vi "TurboMotor.vi"() -> ()   [LabVIEW 2011]
panel:
  in  "Attribute Message Types":u16(ring) items=["Position Control Supervisor"=26, "Position Controller"=27]
  in  "Position Controller Supervisor":u16(ring) items=["Number of Attributes"=1, "Attribute List"=2, "Mode"=3, "Target Position"=6, "Target Velocity"=7, "Acceleration"=8, "Incremental Position Flag"=10, "Load Data/Start Profile/Profile in Progress"=11, "Actual Position"=13, "Actual Velocity"=14, "Commanded Position"=15, "Commanded Velocity"=16, "Enable"=17, "Smooth Stop"=20, "Hard Stop"=21, "Direction"=23, "Reference Direction"=24, "Torque"=25, "Wrap Around"=29, "Kp"=30, "Ki"=31, "Kd"=32, "MaxKi"=33, "Velocity Feed Forward"=35, "Sample Rate"=37, "Feedback Resolution"=40, ""=41, ""=42, ""=43, ""=44, "Max Dynamic Following Error"=45, "Following Error Fault"=47, "Actual Following Error"=48, "Hard Limit Action"=49, "Forward Limit"=50, "Reverse Limit"=51, "Soft Limits Enable"=52, "Soft Limit Action"=53, "Positive Soft Limit Position"=54, "Negative Soft Limit Position"=55, "Positive Limit Triggered"=56, "Negative Limit Triggered"=57, "Load Data Complete"=58, "Current Limit"=100, "Reset Motor Faults"=101, "Reset Motor"=102, "Overheat Setpoint"=103, "Temperature"=104, "Variable u"=105, "Variable v"=106, "Variable w"=107, "Variable x"=108, "GOSUBnnn"=109, "Loss of Network Action"=110, "Status Word"=111]
  in  "stop":bool
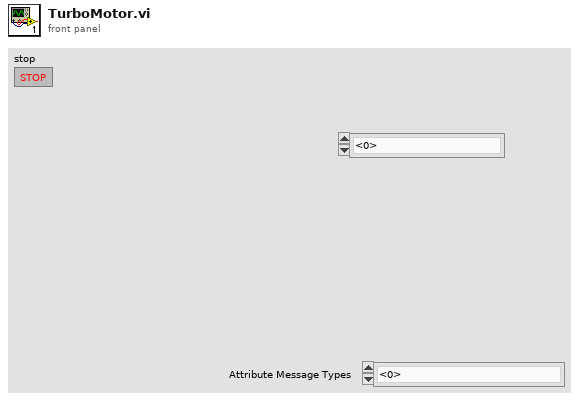
[diagram p1: front panel]
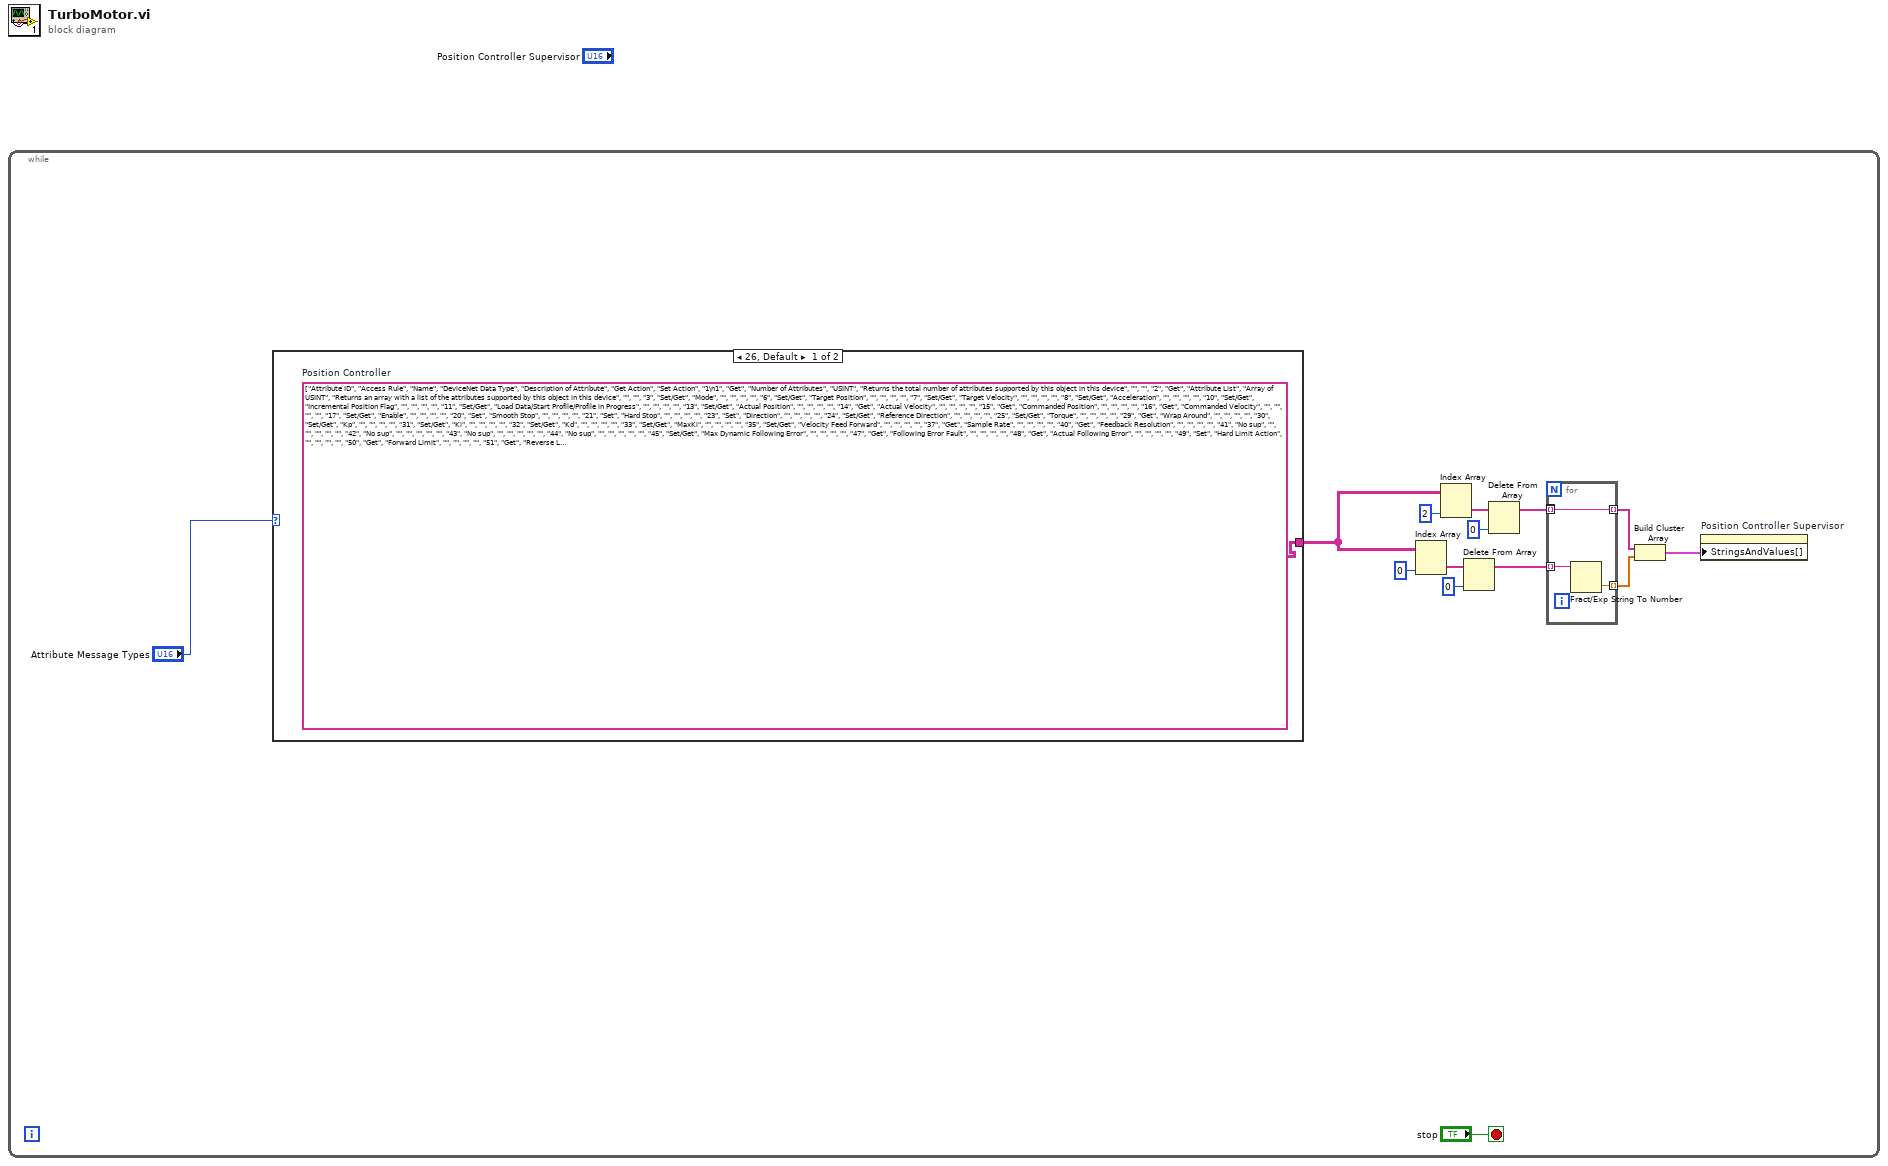
[diagram p0: block diagram]
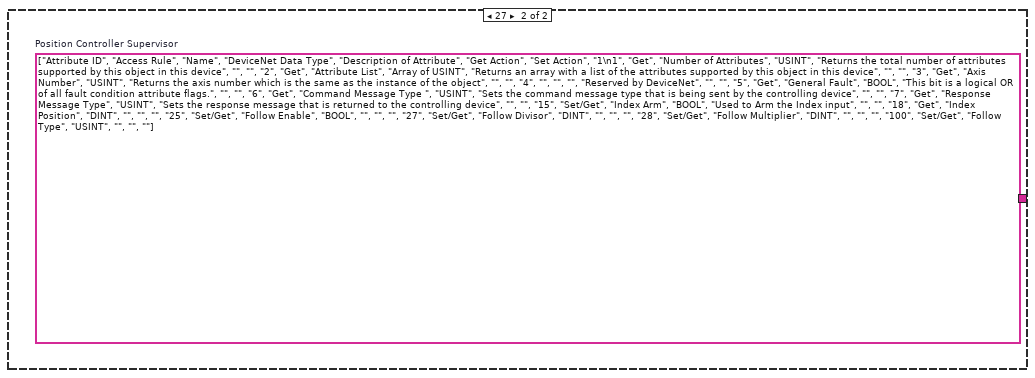
[diagram p2: hidden frame]
diagram:
  n1 = while {
    stop <- "stop" stop-if-true
    n2 = case shown="26, Default" "Attribute Message Types" {
      tunnel: [w15 w16] -> w3
      frame 26, Default {
        w15 = string[][] [["Attribute ID", "Access Rule", "Name", "DeviceNet Data Type", "Description of Attribute", "Get Action", "Set Action"], ["1\n1", "Get", "Number of Attributes", "USINT", "Returns the total number of attributes supported by this object in this device", "", ""], ["2", "Get", "Attribute List", "Array of USINT", "Returns an array with a list of the attributes supported by this object in this device", "", ""], ["3", "Set/Get", "Mode", "", "", "", ""], ["6", "Set/Get", "Target Position", "", "", "", ""], ["7", "Set/Get", "Target Velocity", "", "", "", ""], ["8", "Set/Get", "Acceleration", "", "", "", ""], ["10", "Set/Get", "Incremental Position Flag", "", "", "", ""], ["11", "Set/Get", "Load Data/Start Profile/Profile in Progress", "", "", "", ""], ["13", "Set/Get", "Actual Position", "", "", "", ""], ["14", "Get", "Actual Velocity", "", "", "", ""], ["15", "Get", "Commanded Position", "", "", "", ""], ["16", "Get", "Commanded Velocity", "", "", "", ""], ["17", "Set/Get", "Enable", "", "", "", ""], ["20", "Set", "Smooth Stop", "", "", "", ""], ["21", "Set", "Hard Stop", "", "", "", ""], ["23", "Set", "Direction", "", "", "", ""], ["24", "Set/Get", "Reference Direction", "", "", "", ""], ["25", "Set/Get", "Torque", "", "", "", ""], ["29", "Get", "Wrap Around", "", "", "", ""], ["30", "Set/Get", "Kp", "", "", "", ""], ["31", "Set/Get", "Ki", "", "", "", ""], ["32", "Set/Get", "Kd", "", "", "", ""], ["33", "Set/Get", "MaxKi", "", "", "", ""], ["35", "Set/Get", "Velocity Feed Forward", "", "", "", ""], ["37", "Get", "Sample Rate", "", "", "", ""], ["40", "Get", "Feedback Resolution", "", "", "", ""], ["41", "No sup", "", "", "", "", ""], ["42", "No sup", "", "", "", "", ""], ["43", "No sup", "", "", "", "", ""], ["44", "No sup", "", "", "", "", ""], ["45", "Set/Get", "Max Dynamic Following Error", "", "", "", ""], ["47", "Get", "Following Error Fault", "", "", "", ""], ["48", "Get", "Actual Following Error", "", "", "", ""], ["49", "Set", "Hard Limit Action", "", "", "", ""], ["50", "Get", "Forward Limit", "", "", "", ""], ["51", "Get", "Reverse Limit", "", "", "", ""], ["52", "Set/Get", "Soft Limits Enable", "", "", "", ""], ["53", "Set/Get", "Soft Limit Action", "", "", "", ""], ["54", "Set/Get", "Positive Soft Limit Position", "", "", "", ""], ["55", "Set/Get", "Negative Soft Limit Position", "", "", "", ""], ["56", "Get", "Positive Limit Triggered", "", "", "", ""], ["57", "Get", "Negative Limit Triggered", "", "", "", ""], ["58", "Get", "Load Data Complete", "", "", "", ""], ["100", "Set", "Current Limit", "", "", "", ""], ["101", "Set", "Reset Motor Faults", "", "", "", ""], ["102", "Set", "Reset Motor", "", "", "", ""], ["103", "Set/Get", "Overheat Setpoint", "", "", "", ""], ["104", "Get", "Temperature", "", "", "", ""], ["105", "Set/Get", "Variable u", "", "", "", ""], ["106", "Set/Get", "Variable v", "", "", "", ""], ["107", "Set/Get", "Variable w", "", "", "", ""], ["108", "Set/Get", "Variable x", "", "", "", ""], ["109", "Set", "GOSUBnnn", "", "", "", ""], ["110", "Get", "Loss of Network Action", "", "", "", ""], ["111", "Get", "Status Word", "", "", "", ""]]  # Position Controller
      }
      frame 27 {
        w16 = string[][] [["Attribute ID", "Access Rule", "Name", "DeviceNet Data Type", "Description of Attribute", "Get Action", "Set Action"], ["1\n1", "Get", "Number of Attributes", "USINT", "Returns the total number of attributes supported by this object in this device", "", ""], ["2", "Get", "Attribute List", "Array of USINT", "Returns an array with a list of the attributes supported by this object in this device", "", ""], ["3", "Get", "Axis Number", "USINT", "Returns the axis number which is the same as the instance of the object", "", ""], ["4", "", "", "", "Reserved by DeviceNet", "", ""], ["5", "Get", "General Fault", "BOOL", "This bit is a logical OR of all fault condition attribute flags.", "", ""], ["6", "Get", "Command Message Type ", "USINT", "Sets the command message type that is being sent by the controlling device", "", ""], ["7", "Get", "Response Message Type", "USINT", "Sets the response message that is returned to the controlling device", "", ""], ["15", "Set/Get", "Index Arm", "BOOL", "Used to Arm the Index input", "", ""], ["18", "Get", "Index Position", "DINT", "", "", ""], ["25", "Set/Get", "Follow Enable", "BOOL", "", "", ""], ["27", "Set/Get", "Follow Divisor", "DINT", "", "", ""], ["28", "Set/Get", "Follow Multiplier", "DINT", "", "", ""], ["100", "Set/Get", "Follow Type", "USINT", "", "", ""]]  # Position Controller Supervisor
      }
    }
    n3 = Index Array(array=w3, index (col)=0 ("disabled index (col)")) -> (element=w9:string[])  [unwired: 1 in]
    n4 = Index Array(array=w3, index (col)=2 ("disabled index (col)")) -> (element=w12:string[])  [unwired: 1 in]
    n5 = Delete From Array(array=w9, index=0) -> (array with subset deleted=w7:string[])  [unwired: 1 in, 1 out]
    n6 = Delete From Array(array=w12, index=0) -> (array with subset deleted=w6:string[])  [unwired: 1 in, 1 out]
    n7 = for {
      tunnel: w7 -> [w19] mode=indexing
      tunnel: [w18] -> _ mode=indexing
      tunnel: w6 -> [w18] mode=indexing
      tunnel: [w18] -> w5 mode=indexing
      tunnel: [w17] -> w4 mode=indexing
      n8 = Fract/Exp String To Number(string=w19) -> (number=w17:dbl)  [unwired: 3 in, 1 out]
    }
    n9 = Build Cluster Array(w5, w4) -> (w2:cluster{string, dbl}[])
    n10 = property on="Position Controller Supervisor" class="Ring (strict)"("StringsAndValues[]"=w2) -> ()  [unwired: 2 in, 2 out]
  }
